vi "Sweep control.vi"(0 "Scan control":cluster{"Priority":u16, "Scan name":u16}[](array[cluster])=[{"Priority"=0, "Scan name"=1}, {"Priority"=3, "Scan name"=0}, {"Priority"=2, "Scan name"=0}, {"Priority"=1, "Scan name"=5}] {"Scan name" items=["OFF", "Vsg1", "Vsg2", "Vsgw", "Vbg", "Field", "Temp"]; "Priority" items=["Priority 0", "Priority 1", "Priority 2", "Priority 3", "Priority 4", "Priority 5"]}, 1 "Scan parameters":T2(array[cluster])=[{"DAQ Channel"=1, "Label"="\nappliedVsg=", "Scaled low"=-0.1, "Scaled high"=0.1, "Start"=0.0, "End"=0.18, "Step"=0.0001, "Scale?"=FALSE}, {"DAQ Channel"=2, "Label"="\nappliedTemperature=", "Scaled low"=-0.175, "Scaled high"=0.775, "Start"=0.1, "End"=0.9, "Step"=0.1, "Scale?"=FALSE}, {"DAQ Channel"=3, "Label"="\nappliedVbg=", "Scaled low"=-0.11, "Scaled high"=0.31, "Start"=-0.5, "End"=0.5, "Step"=0.001, "Scale?"=FALSE}, {"DAQ Channel"=3, "Label"="\nappliedField=", "Scaled low"=-0.060000000000000005, "Scaled high"=0.14, "Start"=-10000.0, "End"=0.0, "Step"=2000.0, "Scale?"=FALSE}] {"Step" format="%#_6f"; "End" format="%#_6f"; "Start" format="%#_6f"; "Scaled high" format="%#_6p"; "Scaled low" format="%#_6p"}, 2 "OSC Configuration":T1(array[cluster])=[{"Signal Type"=enum."Sawtooth Wave", "DC"=0.00034, "Amplitude"=0.0015, "frequency"=0.4, "Phase"=180.0}, {"Signal Type"=enum."Sine Wave", "DC"=0.0, "Amplitude"=0.0, "frequency"=1.0, "Phase"=0.0}, {"Signal Type"=enum."Sine Wave", "DC"=0.0, "Amplitude"=0.0, "frequency"=1.0, "Phase"=0.0}, {"Signal Type"=enum."Sine Wave", "DC"=0.0, "Amplitude"=0.0, "frequency"=1.0, "Phase"=0.0}] {"frequency" format="%0.2p"; "Amplitude" format="%0.2p"; "DC" format="%.2p"}, 3 "Comments":string="SA02704G.20140716\nbackgate=0V", 4 "Experiment folder name":string="3- sweep Vsg_50mK_field", 8 "Additional action (indexing priority)":u16[](array[ring])=[4, 2, 4, 4] items=["Clear DAQ Tasks", "Check Temperature", "Check Field Value", "Wait", "Do Nothing"]) -> ()   [LabVIEW 2013]
uses:
  lockin/branches/PPMS-demomode-JL/Lockin-4461_MultiChannel - IV 3.0 globals.vi
panel:
  in  "Number of IV curves":i32=1
  # "Instructions: \n1, you can put multiple scan names in one priority.\n2 OFF has to put in last priority"
  # "I wanted to check the temperature as well as the field (so the zero-field data isn't taken at higher temperatures) so I changed the post-action subvi slightly. In the 'check temperature' case, I made the stop condition that the temp is less than 70mK. By putting 'check temperature' with priority 1, i figure it'll set Vsg1&2 at 0, then wait for the temp to reach 70mK, before it starts sweeping prioity 0."
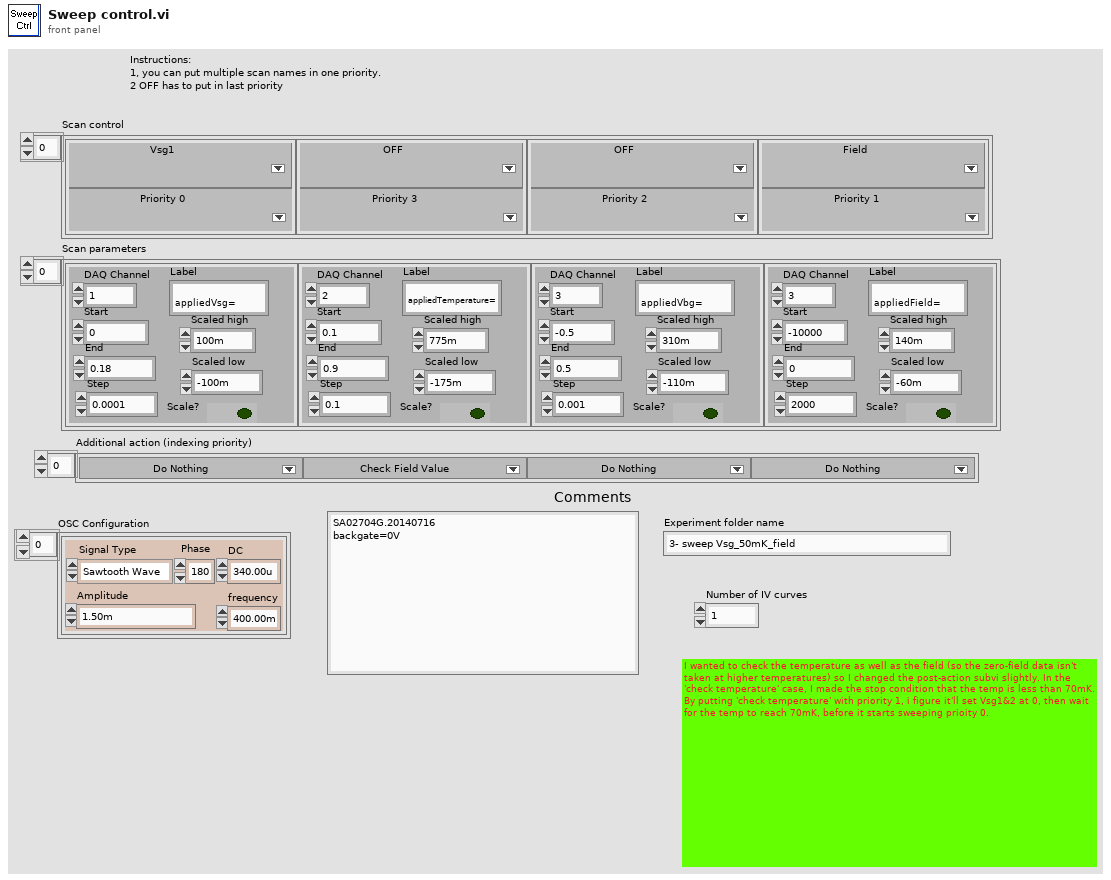
[diagram p1: front panel]
types:
  T1 = cluster{"Signal Type":enum16{"Sine Wave", "Triangle Wave", "Square Wave", "Sawtooth Wave"}, "DC":dbl, "Amplitude":dbl, "frequency":dbl, "Phase":dbl}[]
  T2 = cluster{"DAQ Channel":i32, "Label":string, "Scaled low":dbl, "Scaled high":dbl, "Start":dbl, "End":dbl, "Step":dbl, "Scale?":bool}[]
  T3 = cluster{cluster{"DAQ Channel":i32, "Label":string, "Scaled low":dbl, "Scaled high":dbl, "Start":dbl, "End":dbl, "Step":dbl, "Scale?":bool}[]}[]
  T4 = cluster{cluster{"Priority":u16, "Scan name":u16}[]}[]
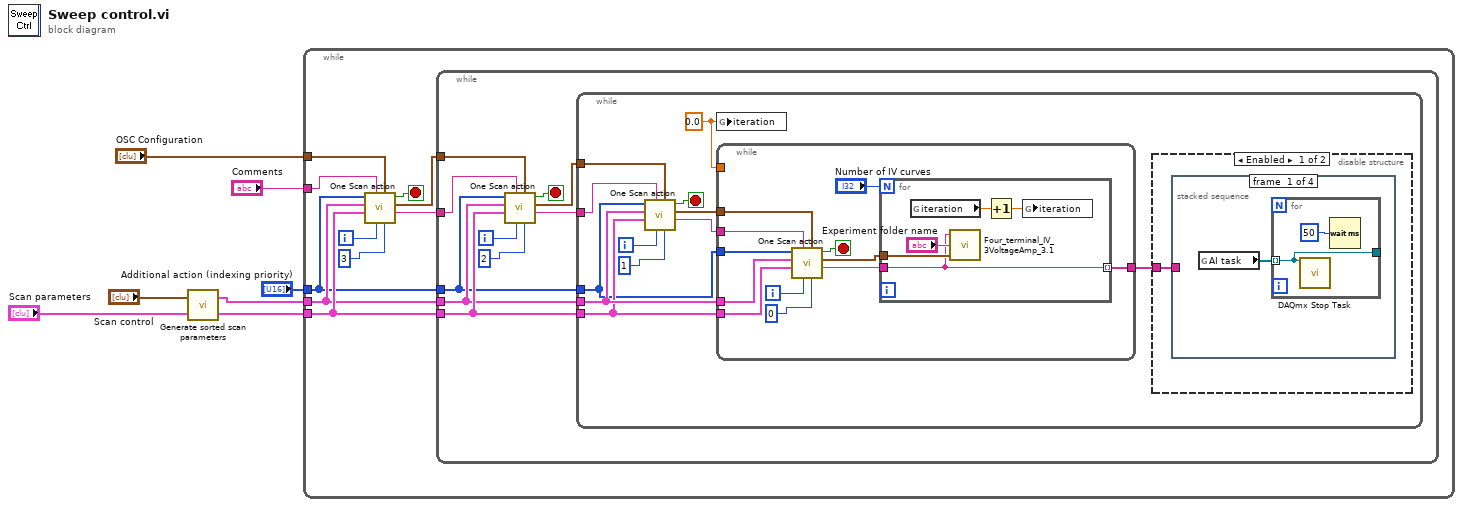
[diagram p0: block diagram]
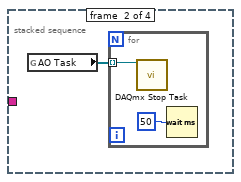
[diagram p2: hidden frame]
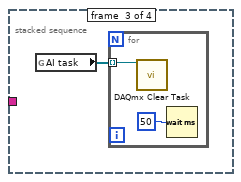
[diagram p3: hidden frame]
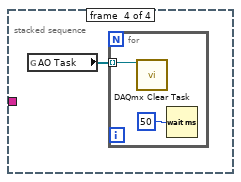
[diagram p4: hidden frame]
diagram:
  n1 = call "Generate sorted scan parameters.vi"("Scan parameters"="Scan parameters", "Scan control"="Scan control") -> ("Sorted scan parameters"=w3:T3, "Sorted scan control"=w2:T4)
  n2 = while {
    tunnel: "Comments" -> [w12]
    tunnel: "OSC Configuration" -> [w13]
    tunnel: w3 -> [w17]
    tunnel: w2 -> [w16]
    tunnel: "Additional action (indexing priority)" -> [w14]
    i -> [w8]
    stop <- w15 stop-if-true
    n3 = call "One Scan action.vi"("Action"=3, "OSC Configuration in"=w13, "index"=w8, "Comments in"=w12, "Sorted scan parameters"=w17, "Sorted scan control"=w16, "Additional action (indexing priority)"=w14) -> ("Comments out"=w10:string, "OSC Configuration out"=w11:T1, "Stop?"=w15:bool)  [unwired: 2 in]
    n4 = while {
      tunnel: w17 -> [w27]
      tunnel: w16 -> [w26]
      tunnel: w14 -> [w25]
      tunnel: w10 -> [w24]
      tunnel: w11 -> [w23]
      i -> [w18]
      stop <- w22 stop-if-true
      n5 = call "One Scan action.vi"("Action"=2, "OSC Configuration in"=w23, "index"=w18, "Comments in"=w24, "Sorted scan parameters"=w27, "Sorted scan control"=w26, "Additional action (indexing priority)"=w25) -> ("Comments out"=w20:string, "OSC Configuration out"=w21:T1, "Stop?"=w22:bool)  [unwired: 2 in]
      n6 = while {
        tunnel: w21 -> [w37]
        tunnel: w20 -> [w36]
        tunnel: w26 -> [w35]
        tunnel: w27 -> [w34]
        tunnel: w25 -> [w33]
        i -> [w29]
        stop <- w30 stop-if-true
        w39 = 0.0 ("iteration")
        n7 = call "One Scan action.vi"("Action"=1, "OSC Configuration in"=w37, "index"=w29, "Comments in"=w36, "Sorted scan parameters"=w34, "Sorted scan control"=w35, "Additional action (indexing priority)"=w33) -> ("Comments out"=w32:string, "OSC Configuration out"=w31:T1, "Stop?"=w30:bool)  [unwired: 2 in]
        n8 = global write "Lockin-4461_MultiChannel - IV 3.0 globals.vi" "iteration"(w39) -> ()
        n9 = while {
          tunnel: w35 -> [w63]
          tunnel: w34 -> [w62]
          tunnel: w31 -> [w61]
          tunnel: w32 -> [w60]
          tunnel: w33 -> [w56]
          tunnel: w39 -> [_]
          tunnel: [w55] -> w38
          i -> [w53]
          stop <- w57 stop-if-true
          n10 = call "One Scan action.vi"("Action"=0, "OSC Configuration in"=w61, "index"=w53, "Comments in"=w60, "Sorted scan parameters"=w62, "Sorted scan control"=w63, "Additional action (indexing priority)"=w56) -> ("Comments out"=w58:string, "OSC Configuration out"=w59:T1, "Stop?"=w57:bool)  [unwired: 2 in]
          n11 = for {
            N: "Number of IV curves" -> [_]
            tunnel: w59 -> [w68]
            tunnel: w58 -> [w67]
            tunnel: [w67] -> w55 mode=indexing
            n12 = global read "Lockin-4461_MultiChannel - IV 3.0 globals.vi" "iteration"() -> (w66:dbl)
            n13 = call "Four_terminal_IV_3VoltageAmp_3.1.vi"("Comments"=w67, "Experiment folder name"="Experiment folder name", "OSC Configuration"=w68) -> ()  [unwired: 1 in, 5 out]
            n14 = Increment(x=w66) -> (x+1=w65:dbl)
            n15 = global write "Lockin-4461_MultiChannel - IV 3.0 globals.vi" "iteration"(w65) -> ()
          }
        }
        n16 = disable-structure shown="Enabled" {
          disable-tunnel: w38 -> [w40 _]
          frame Enabled {
            n17 = stacked-sequence {
              tunnel: w40 -> [_ _ _ _]
              frame #0 {
                n18 = global read "Lockin-4461_MultiChannel - IV 3.0 globals.vi" "AI task"() -> (w41:refnum<k21>[])
                n19 = for {
                  tunnel: w41 -> [w42] mode=indexing
                  tunnel: [w42] -> _
                  n20 = call <vilib>:"DAQmx Stop Task.vi"("task/channels in"=w42) -> ()  [unwired: 13 in, 2 out]
                  n21 = Wait (ms)(milliseconds to wait=u32 50) -> ()  [unwired: 1 out]
                }
              }
              frame #1 {
                n22 = global read "Lockin-4461_MultiChannel - IV 3.0 globals.vi" "AO Task"() -> (w44:refnum<k21>[])
                n23 = for {
                  tunnel: w44 -> [w46] mode=indexing
                  n24 = call <vilib>:"DAQmx Stop Task.vi"("task/channels in"=w46) -> ()  [unwired: 13 in, 2 out]
                  n25 = Wait (ms)(milliseconds to wait=u32 50) -> ()  [unwired: 1 out]
                }
              }
              frame #2 {
                n26 = global read "Lockin-4461_MultiChannel - IV 3.0 globals.vi" "AI task"() -> (w47:refnum<k21>[])
                n27 = for {
                  tunnel: w47 -> [w49] mode=indexing
                  n28 = call <vilib>:"DAQmx Clear Task.vi"("task in"=w49) -> ()  [unwired: 14 in, 1 out]
                  n29 = Wait (ms)(milliseconds to wait=u32 50) -> ()  [unwired: 1 out]
                }
              }
              frame #3 {
                n30 = global read "Lockin-4461_MultiChannel - IV 3.0 globals.vi" "AO Task"() -> (w50:refnum<k21>[])
                n31 = for {
                  tunnel: w50 -> [w52] mode=indexing
                  n32 = call <vilib>:"DAQmx Clear Task.vi"("task in"=w52) -> ()  [unwired: 14 in, 1 out]
                  n33 = Wait (ms)(milliseconds to wait=u32 50) -> ()  [unwired: 1 out]
                }
              }
            }
          }
          frame Disabled {
          }
        }
      }
    }
  }
